vi "EditGroup.vi"() -> ()   [LabVIEW 2020, in "Curve Editor.lvlib"]
uses:
  Curve Editor.lvlib
  Key Value/Key Value.lvlib
panel:
  in  "重复":i32=1 min=1
  in  "Tree引用句柄":refnum<vi>
  in  "周期":i32
  in  "索引":i32
  in  "取消按钮":bool
  in  "确定按钮":bool
  in  "组名":string
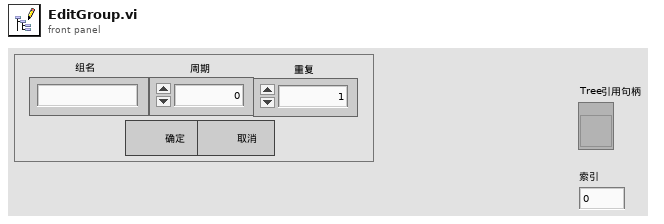
[diagram p1: front panel]
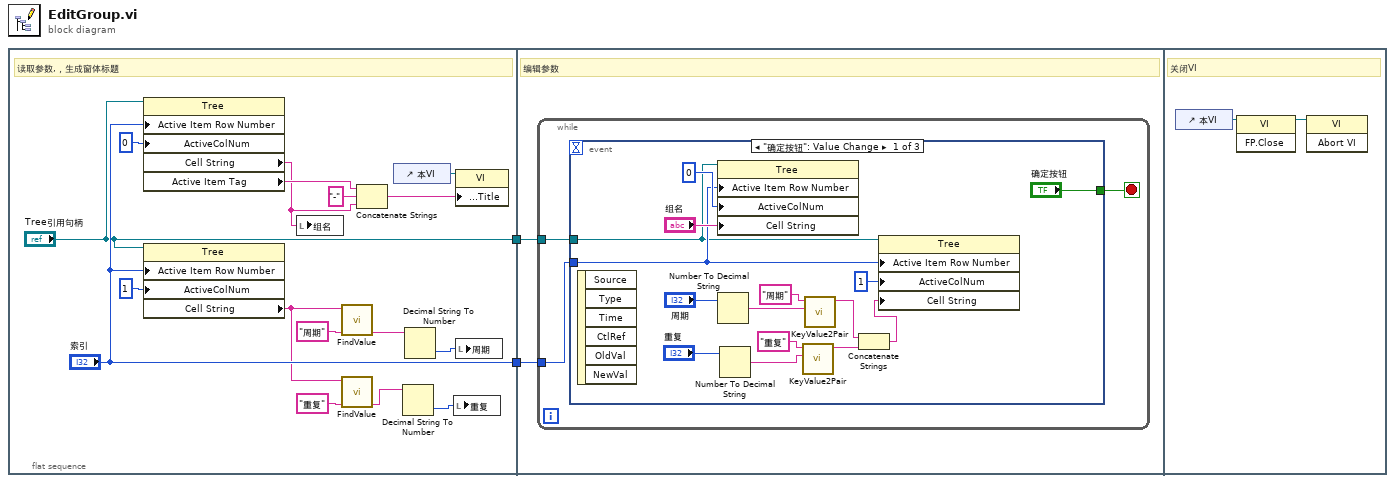
[diagram p0: block diagram]
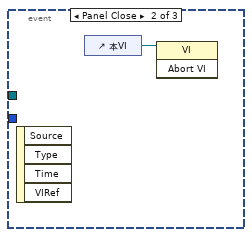
[diagram p2: hidden frame]
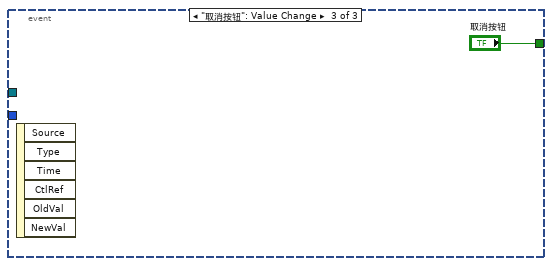
[diagram p3: hidden frame]
diagram:
  n1 = flat-sequence {
    tunnel: ["索引"] -> w2
    tunnel: ["Tree引用句柄"] -> w1
    tunnel: w2 -> [w20]
    tunnel: w1 -> [w19]
    frame #0 {
      # "读取参数,，生成窗体标题"
      n2 = property class="Tree"(reference="Tree引用句柄", "Active Item Row Number"="索引", "ActiveColNum"=0 ("活动单元格:活动列数")) -> ("Cell String"=w8:string, "Active Item Tag"=w10:string)  [unwired: 1 in, 2 out]
      n3 = property class="Tree"(reference="Tree引用句柄", "Active Item Row Number"="索引", "ActiveColNum"=1 ("活动单元格:活动列数")) -> ("Cell String"=w3:string)  [unwired: 1 in, 2 out]
      n4 = local write "组名"(w8) -> ()
      n5 = call "FindValue.vi"("键"="周期", "键值串"=w3) -> ("值"=w14:string)  [unwired: 8 in, 1 out]
      n6 = call "FindValue.vi"("键"="重复", "键值串"=w3) -> ("值"=w4:string)  [unwired: 8 in, 1 out]
      n7 = Concatenate Strings(w10, "-" ("字符串"), w8) -> (w7:string)
      n8 = control-ref of="本VI"() -> (w18:refnum<vi>)
      n9 = Decimal String To Number(string=w4) -> (number=w5:i32)  [unwired: 2 in, 1 out]
      n10 = Decimal String To Number(string=w14) -> (number=w13:i32)  [unwired: 2 in, 1 out]
      n11 = local write "重复"(w5) -> ()
      n12 = property class="VI"(reference=w18, "Front Panel.Title"=w7) -> ()  [unwired: 1 in, 2 out]
      n13 = local write "周期"(w13) -> ()
    }
    frame #1 {
      # "编辑参数"
      n14 = while {
        tunnel: w20 -> [w22]
        tunnel: w19 -> [w21]
        stop <- w23 stop-if-true
        n15 = event shown="[0] \"确定按钮\": Value Change" {
          selector: _ -> [_ _ _]
          dyn-events: _ -> [_ _ _]
          timeout: _ -> [_ _ _]
          tunnel: ["确定按钮" _ "取消按钮"] -> w23
          tunnel: w22 -> [w32 _ _]
          tunnel: w21 -> [w30 _ _]
          event "确定按钮": Value Change {
            n16 = event-data() -> ()  [unwired: 1 in, 6 out]
            n17 = property class="Tree"(reference=w30, "Active Item Row Number"=w32, "ActiveColNum"=0 ("活动单元格:活动列数"), "Cell String"="组名") -> ()  [unwired: 1 in, 2 out]
            n18 = Number To Decimal String(number="周期") -> (decimal integer string=w35:string)  [unwired: 1 in]
            n19 = Number To Decimal String(number="重复") -> (decimal integer string=w27:string)  [unwired: 1 in]
            n20 = call "KeyValue2Pair.vi"("值"=w27, "键"="重复") -> ("键值对"=w26:string)  [unwired: 9 in]
            n21 = call "KeyValue2Pair.vi"("值"=w35, "键"="周期") -> ("键值对"=w25:string)  [unwired: 9 in]
            n22 = Concatenate Strings(w25, w26) -> (w24:string)
            n23 = property class="Tree"(reference=w30, "Active Item Row Number"=w32, "ActiveColNum"=1 ("活动单元格:活动列数"), "Cell String"=w24) -> ()  [unwired: 1 in, 2 out]
          }
          event Panel Close {
            n24 = event-data() -> ()  [unwired: 1 in, 4 out]
            n25 = control-ref of="本VI"() -> (w39:refnum<vi>)
            n26 = invoke class="VI" method="Abort VI"(reference=w39) -> ()  [unwired: 2 in, 3 out]
          }
          event "取消按钮": Value Change {
            n27 = event-data() -> ()  [unwired: 1 in, 6 out]
          }
        }
      }
    }
    frame #2 {
      # "关闭VI"
      n28 = control-ref of="本VI"() -> (w42:refnum<vi>)
      n29 = invoke class="VI" method="FP.Close"(reference=w42) -> (reference out=w41:refnum<vi>)  [unwired: 2 in, 2 out]
      n30 = invoke class="VI" method="Abort VI"(reference=w41) -> ()  [unwired: 2 in, 3 out]
    }
  }
